vi "NewAutoRelTrajSelector.vi"(11 "RelativeTrajectoryInput":i32) -> (3 "RelativeTrajectoryOutput":T1 {"States"."POSE"."ROTATION"."SIN" format="%13.4f"; "States"."POSE"."ROTATION"."COS" format="%13.4f"; "States"."POSE"."ROTATION"."VALUE" format="%13.4f"; "States"."POSE"."TRANSLATION"."Y" format="%14.3f"; "States"."POSE"."TRANSLATION"."X" format="%14.3f"; "TotalTImeSecs" format="%20.3f"})   [LabVIEW 2023]
uses:
  Trajectory/TrajectoryGlobals.vi
  <vilib>/Rock Robotics/WPI/ThirdParty/JAS_Junk/TrajLib/TypeDef/TRANSLATION2D.ctl
  <vilib>/Rock Robotics/WPI/ThirdParty/JAS_Junk/TrajLib/Trajectory_Library.lvlib
  <vilib>/Rock Robotics/WPI/ThirdParty/JAS_Junk/TrajLib/TypeDef/ROTATION2D.ctl
  <vilib>/Rock Robotics/WPI/ThirdParty/JAS_Junk/TrajLib/TypeDef/POSE2D.ctl
  <vilib>/Rock Robotics/WPI/ThirdParty/JAS_Junk/TrajLib/TypeDef/TRAJ_STATE.ctl
  <vilib>/Rock Robotics/WPI/ThirdParty/JAS_Junk/TrajLib/TypeDef/TRAJECTORY.ctl
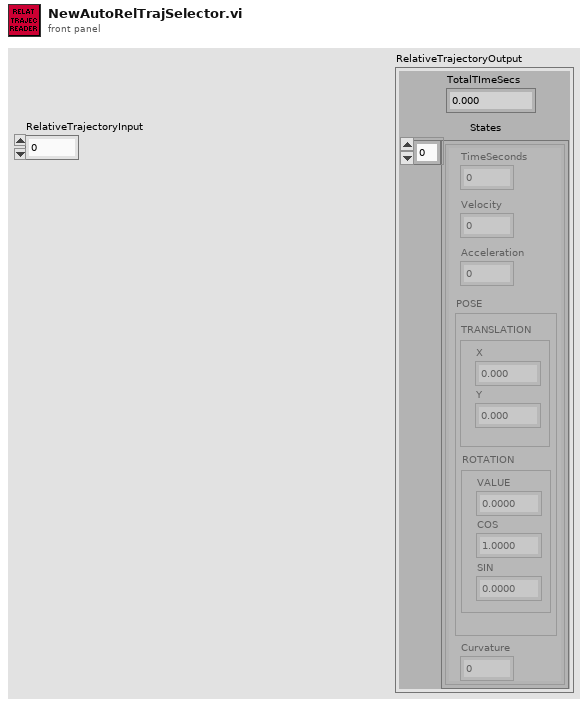
[diagram p1: front panel]
types:
  T1 = typedef "Trajectory_Library.lvlib/TRAJECTORY.ctl" = cluster{"TotalTImeSecs":dbl, "States":T2[]}
  T2 = typedef "Trajectory_Library.lvlib/TRAJ_STATE.ctl" = cluster{"TimeSeconds":dbl, "Velocity":dbl, "Acceleration":dbl, "POSE":T3, "Curvature":dbl}
  T3 = typedef "Trajectory_Library.lvlib/POSE2D.ctl" = cluster{"TRANSLATION":T4, "ROTATION":T5}
  T4 = typedef "Trajectory_Library.lvlib/TRANSLATION2D.ctl" = cluster{"X":dbl, "Y":dbl}
  T5 = typedef "Trajectory_Library.lvlib/ROTATION2D.ctl" = cluster{"VALUE":dbl, "COS":dbl, "SIN":dbl}
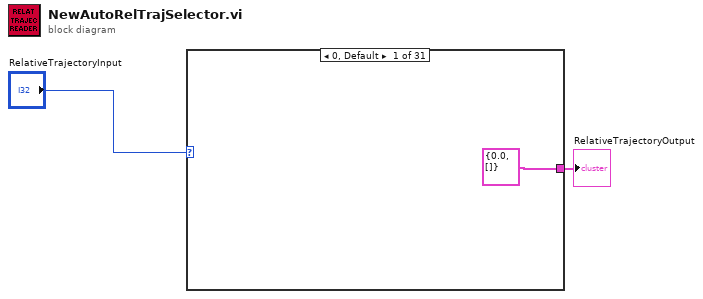
[diagram p0: block diagram]
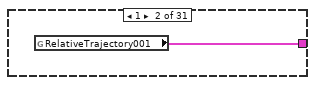
[diagram p2: hidden frame]
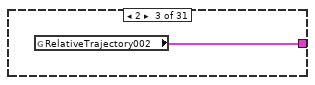
[diagram p3: hidden frame]
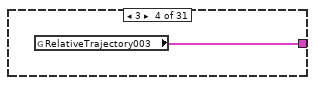
[diagram p4: hidden frame]
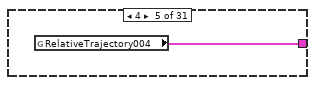
[diagram p5: hidden frame]
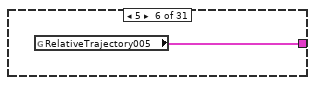
[diagram p6: hidden frame]
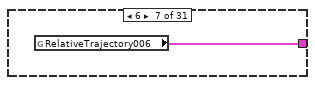
[diagram p7: hidden frame]
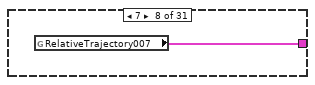
[diagram p8: hidden frame]
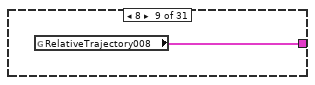
[diagram p9: hidden frame]
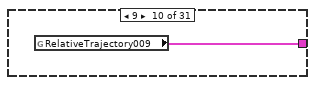
[diagram p10: hidden frame]
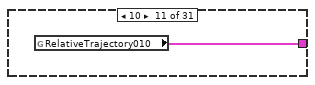
[diagram p11: hidden frame]
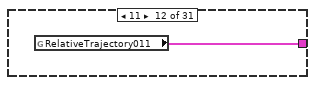
[diagram p12: hidden frame]
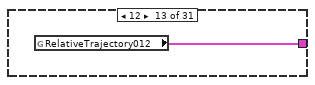
[diagram p13: hidden frame]
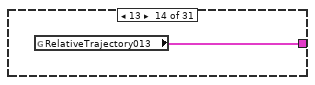
[diagram p14: hidden frame]
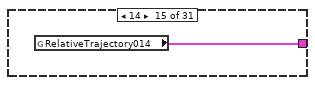
[diagram p15: hidden frame]
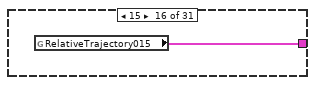
[diagram p16: hidden frame]
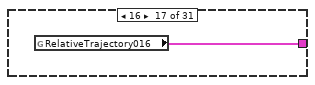
[diagram p17: hidden frame]
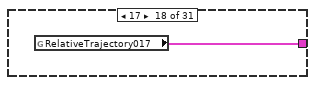
[diagram p18: hidden frame]
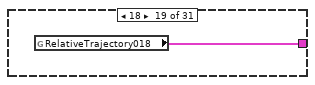
[diagram p19: hidden frame]
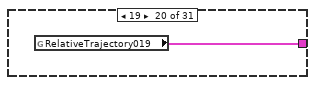
[diagram p20: hidden frame]
diagram:
  n1 = case shown="0, Default" "RelativeTrajectoryInput" {
    tunnel: [T1 {"TotalTImeSecs"=0.0, "States"=[]} ("RelativeTrajectory001") w4 w5 w6 w7 w8 w9 w10 w11 w12 w13 w14 w15 w16 w17 w18 w19 w20 w21 w22 w23 w24 w25 w26 w27 w28 w29 w30 w31 w32 w33] -> w1
    frame 0, Default {
    }
    frame 1 {
      n2 = global read "TrajectoryGlobals.vi" "RelativeTrajectory001"() -> (w4:T1)
    }
    frame 2 {
      n3 = global read "TrajectoryGlobals.vi" "RelativeTrajectory002"() -> (w5:T1)
    }
    frame 3 {
      n4 = global read "TrajectoryGlobals.vi" "RelativeTrajectory003"() -> (w6:T1)
    }
    frame 4 {
      n5 = global read "TrajectoryGlobals.vi" "RelativeTrajectory004"() -> (w7:T1)
    }
    frame 5 {
      n6 = global read "TrajectoryGlobals.vi" "RelativeTrajectory005"() -> (w8:T1)
    }
    frame 6 {
      n7 = global read "TrajectoryGlobals.vi" "RelativeTrajectory006"() -> (w9:T1)
    }
    frame 7 {
      n8 = global read "TrajectoryGlobals.vi" "RelativeTrajectory007"() -> (w10:T1)
    }
    frame 8 {
      n9 = global read "TrajectoryGlobals.vi" "RelativeTrajectory008"() -> (w11:T1)
    }
    frame 9 {
      n10 = global read "TrajectoryGlobals.vi" "RelativeTrajectory009"() -> (w12:T1)
    }
    frame 10 {
      n11 = global read "TrajectoryGlobals.vi" "RelativeTrajectory010"() -> (w13:T1)
    }
    frame 11 {
      n12 = global read "TrajectoryGlobals.vi" "RelativeTrajectory011"() -> (w14:T1)
    }
    frame 12 {
      n13 = global read "TrajectoryGlobals.vi" "RelativeTrajectory012"() -> (w15:T1)
    }
    frame 13 {
      n14 = global read "TrajectoryGlobals.vi" "RelativeTrajectory013"() -> (w16:T1)
    }
    frame 14 {
      n15 = global read "TrajectoryGlobals.vi" "RelativeTrajectory014"() -> (w17:T1)
    }
    frame 15 {
      n16 = global read "TrajectoryGlobals.vi" "RelativeTrajectory015"() -> (w18:T1)
    }
    frame 16 {
      n17 = global read "TrajectoryGlobals.vi" "RelativeTrajectory016"() -> (w19:T1)
    }
    frame 17 {
      n18 = global read "TrajectoryGlobals.vi" "RelativeTrajectory017"() -> (w20:T1)
    }
    frame 18 {
      n19 = global read "TrajectoryGlobals.vi" "RelativeTrajectory018"() -> (w21:T1)
    }
    frame 19 {
      n20 = global read "TrajectoryGlobals.vi" "RelativeTrajectory019"() -> (w22:T1)
    }
    frame 20 {
      n21 = global read "TrajectoryGlobals.vi" "RelativeTrajectory020"() -> (w23:T1)
    }
    frame 21 {
      n22 = global read "TrajectoryGlobals.vi" "RelativeTrajectory021"() -> (w24:T1)
    }
    frame 22 {
      n23 = global read "TrajectoryGlobals.vi" "RelativeTrajectory022"() -> (w25:T1)
    }
    frame 23 {
      n24 = global read "TrajectoryGlobals.vi" "RelativeTrajectory023"() -> (w26:T1)
    }
    frame 24 {
      n25 = global read "TrajectoryGlobals.vi" "RelativeTrajectory024"() -> (w27:T1)
    }
    frame 25 {
      n26 = global read "TrajectoryGlobals.vi" "RelativeTrajectory025"() -> (w28:T1)
    }
    frame 26 {
      n27 = global read "TrajectoryGlobals.vi" "RelativeTrajectory026"() -> (w29:T1)
    }
    frame 27 {
      n28 = global read "TrajectoryGlobals.vi" "RelativeTrajectory027"() -> (w30:T1)
    }
    frame 28 {
      n29 = global read "TrajectoryGlobals.vi" "RelativeTrajectory028"() -> (w31:T1)
    }
    frame 29 {
      n30 = global read "TrajectoryGlobals.vi" "RelativeTrajectory029"() -> (w32:T1)
    }
    frame 30 {
      n31 = global read "TrajectoryGlobals.vi" "RelativeTrajectory030"() -> (w33:T1)
    }
  }
  "RelativeTrajectoryOutput" <- w1
